vi "Define Test.vi"(8 "error in (no error)":errorcluster, 9 "register caller level (0)":i32, 11 "Label (VI Title)":string) -> (0 "error out":errorcluster, 2 "Properties.Test":refnum<class "Properties.Test.lvclass">)   [LabVIEW 2020, in "Caraya.lvlib" / "Test.lvclass"]
doc: "Registers the calling VI as a test case.\nTest cases contain one or many assertions.\n\nAll assertions called after the Define Test method, and within the same block diagram, will become part of the test."
uses:
  Test.lvclass
  Properties.Test/Properties.Test.lvclass
  C:/projects/caraya/src/classes/Properties/Properties.lvclass
  Test Assert Factory/Test Assert Factory.lvclass
  Caraya.lvlib
  Assert Factory Manager/Assert Factory Manager.lvclass
  Basic Test Manager/Basic Test Manager.lvclass
  Properties/Properties.lvclass
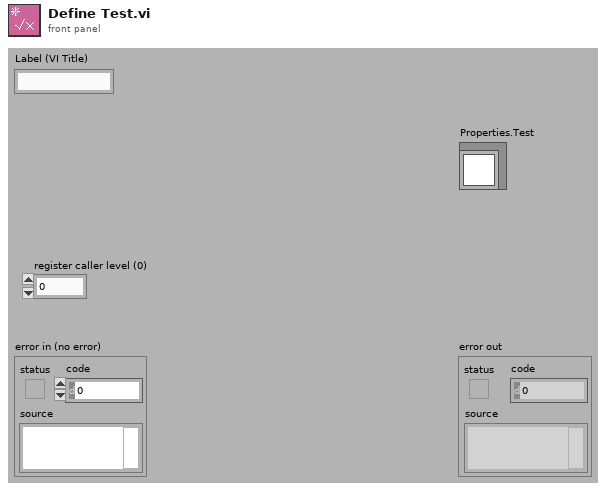
[diagram p1: front panel]
types:
  T1 = typedef "Caraya.lvlib/Test Assert Factory.lvclass/Test Storage -- cluster.ctl" = cluster{"Test UID":string, "Caller UID":string, "Test Label":string, "Call Chain":string[]}
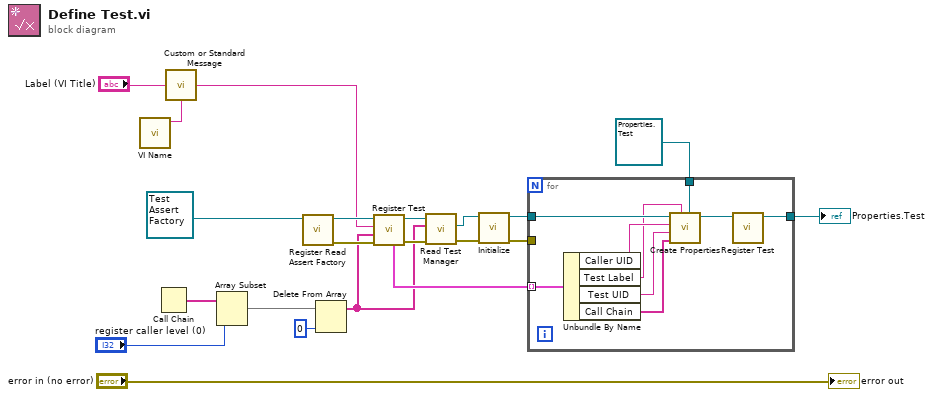
[diagram p0: block diagram]
diagram:
  n1 = call "VI Name.vi"() -> ("VI Name"=w20:string)  [unwired: 10 in, 1 out]
  n2 = Call Chain() -> (call chain=w3:string[])
  n3 = call "Custom or Standard Message.vi"("Custom Message"="Label (VI Title)", "Standard Message"=w20) -> ("Message"=w6:string)
  n4 = Array Subset(array=w3, index="register caller level (0)") -> (w2:string[])  [unwired: 1 in]
  n5 = call "Register Read Assert Factory.vi"("Test Assert Factory"=refnum<class "Test Assert Factory.lvclass"> refnum) -> ("error out"=w11:errorcluster, "Test Assert Factory"=w12:refnum<class "Test Assert Factory.lvclass">)  [unwired: 9 in]
  n6 = Delete From Array(array=w2, index=0) -> (array with subset deleted=w7:string[])  [unwired: 1 in, 1 out]
  n7 = call "Register Test.vi"("error in (no error)"=w11, "VI Call Chain"=w7, "Test Label"=w6, "Assert Factory in"=w12) -> ("error out"=w15:errorcluster, "Assert Factory out"=w16:refnum<class "Test Assert Factory.lvclass">, "Tests to Register"=w10:T1[])  [unwired: 3 in, 2 out]
  n8 = call-dynamic "Read Test Manager.vi"("error in (no error)"=w15, "VI Call Chain"=w7, "Assert Factory in"=w16) -> ("error out"=w18:errorcluster, "Basic Test Manager"=w9:refnum<class "Basic Test Manager.lvclass">)  [unwired: 6 in, 1 out]
  n9 = call "Initialize.vi"("error in (no error)"=w18, "Test Manager in"=w9) -> ("error out"=w14:errorcluster, "Test Manager out"=w8:refnum<class "Basic Test Manager.lvclass">)  [unwired: 8 in]
  n10 = for {
    tunnel: w8 -> [w29]
    tunnel: w14 -> [_]
    tunnel: w10 -> [w30] mode=indexing
    tunnel: refnum<class "Properties.Test.lvclass"> refnum ("Caraya.lvlib:Properties.Test.lvclass") -> [w24]
    tunnel: [w22] -> w4
    n11 = Unbundle By Name(w30) -> ("Caller UID"=w28:string, "Test Label"=w27:string, "Test UID"=w26:string, "Call Chain"=w25:string[])
    n12 = call "Create Properties.vi"("Properties in"=w24, "label"=w27, "call-chain"=w25, "self-id"=w26, "owner-id"=w28, "Test Manager"=w29) -> ("Properties out"=w23:refnum<class "Properties.Test.lvclass">)  [unwired: 5 in]
    n13 = call "Register Test.vi"("Properties.Test in"=w23) -> ("Properties.Test out"=w22:refnum<class "Properties.Test.lvclass">)  [unwired: 10 in]
  }
  "Properties.Test" <- w4
  "error out" <- "error in (no error)"
